vi "H5Gcreate.vi"(2 "name":string, 3 "loc_id":i32, 5 "gapl_id":i32, 7 "gcpl_id":i32, 8 "lcpl_id":u32, 9 "error in (no error)":errorcluster) -> (0 "group_id":i32, 6 "error out":errorcluster)   [LabVIEW 2009]
uses:
  hdf5dll.dll
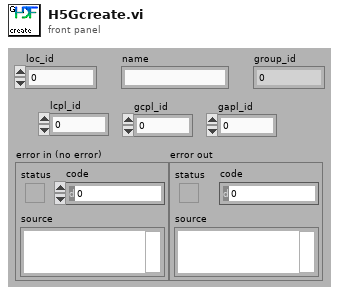
[diagram p1: front panel]
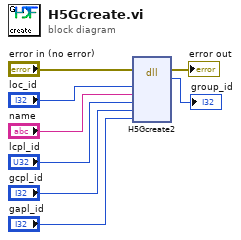
[diagram p0: block diagram]
diagram:
  n1 = dll-call lib="hdf5dll.dll" fn="H5Gcreate2"(error in="error in (no error)", "loc_id"="loc_id", "name"="name", "lcpl_id"="lcpl_id", "gcpl_id"="gcpl_id", "gapl_id"="gapl_id") -> (error out=→"error out":errorcluster, "return type"=→"group_id":i32)  [unwired: 7 in, 1 out]
